vi "Initialize Starter Kit 1.0 (sbRIO-9631).vi"(8 "error in (no error)":errorcluster, 11 "IP address (\"\")":string) -> (0 "error out":errorcluster, 3 "FPGA starter kit host 1.0 out":refnum<class "NI_Robotics_Starter Kit Host_9631_1.0.lvclass">)   [LabVIEW 2017, in "NI_Robotics_Starter Kit Host_9631_1.0.lvclass"]
doc: "Begins a communication session with the FPGA on the robot you want to control and returns a reference you use to read from or write to the FPGA. You must call this VI before you access I/O on the FPGA."
uses:
  <vilib>/robotics/Starter Kit/1.0/9631 Host Interface/NI_Robotics_Starter Kit Host_9631_1.0.lvclass
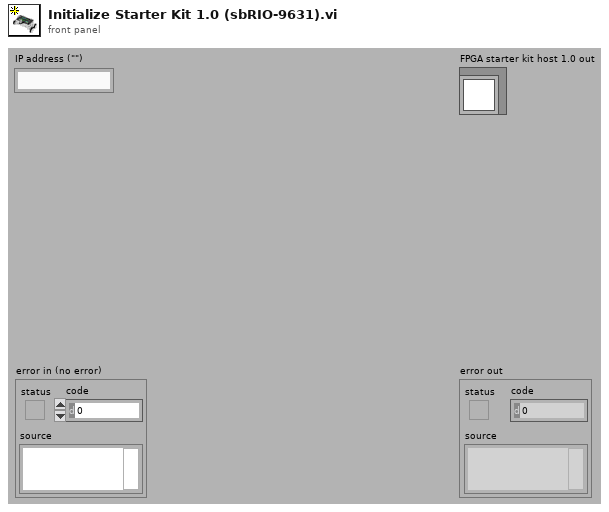
[diagram p1: front panel]
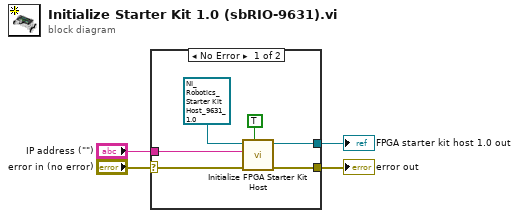
[diagram p0: block diagram]
diagram:
  n1 = case shown="No Error" "error in (no error)" {
    selector: "error in (no error)" -> [w7 w11]
    tunnel: [w6 w11] -> w3
    tunnel: [w8 _] -> w2
    tunnel: "IP address (\"\")" -> [w5 _]
    frame No Error {
      n2 = call-dynamic "Initialize FPGA Starter Kit Host.vi"("run FPGA (T)"=TRUE, "error in (no error)"=w7, "IP address (\"\")"=w5, "FPGA starter kit host in"=refnum<class "NI_Robotics_Starter Kit Host_9631_1.0.lvclass"> refnum ("NI_Robotics_Starter Kit Host_9631_1.0 in")) -> ("error out"=w6:errorcluster, "FPGA starter kit host out"=w8:refnum<class "NI_Robotics_Starter Kit Host_9631_1.0.lvclass">)  [unwired: 6 in]
    }
    frame Error {
    }
  }
  "error out" <- w3
  "FPGA starter kit host 1.0 out" <- w2
